vi "ParamsSenoide.vi"(2 "paramsIn":variant) -> (16 "paramsOut":variant)   [LabVIEW 2017]
uses:
  Typedefs/Tipo_ParamsSenoide.ctl
panel:
  in  "Fase (graus)":dbl
  in  "Frequência (Hz)":dbl
  in  "Init":bool
  in  "Amplitude":dbl
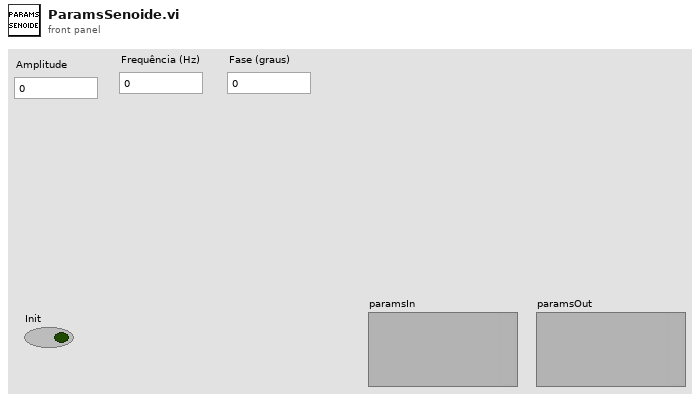
[diagram p1: front panel]
types:
  T1 = typedef "Tipo_ParamsSenoide.ctl" = cluster{"Amplitude":dbl, "Frequencia":dbl, "Fase":dbl}
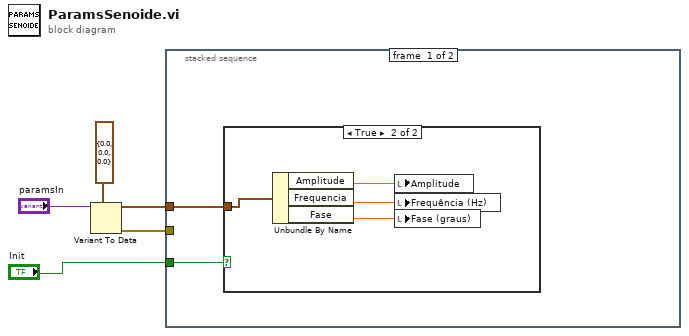
[diagram p0: block diagram]
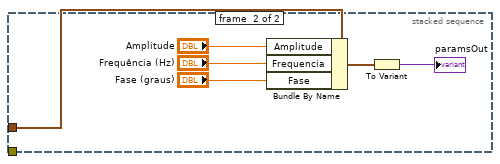
[diagram p3: hidden frame]
diagram:
  n1 = Variant To Data(type=T1 {"Amplitude"=0.0, "Frequencia"=0.0, "Fase"=0.0} ("ParamsIn"), Variant="paramsIn") -> (data=w3:T1, error out=w1:errorcluster)  [unwired: 1 in]
  n2 = stacked-sequence {
    tunnel: w3 -> [w7 w17]
    tunnel: "Init" -> [w6 _]
    tunnel: w1 -> [_ _]
    frame #0 {
      n3 = case shown="True" w6 {
        tunnel: w7 -> [_ w11]
        frame False {
        }
        frame True {
          n4 = Unbundle By Name(w11) -> ("Amplitude"=w10:dbl, "Frequencia"=w9:dbl, "Fase"=w8:dbl)
          n5 = local write "Amplitude"(w10) -> ()
          n6 = local write "Frequência (Hz)"(w9) -> ()
          n7 = local write "Fase (graus)"(w8) -> ()
        }
      }
    }
    frame #1 {
      n8 = Bundle By Name(cluster=w17, "Amplitude"="Amplitude", "Frequencia"="Frequência (Hz)", "Fase"="Fase (graus)") -> (w15:T1)
      n9 = To Variant(anything=w15) -> (Variant=→"paramsOut":variant)
    }
  }
